vi "filter_test.vi"(9 "Throughput-1":i16=17, 10 "reset":bool, 11 "input valid":bool) -> (0 "run?":bool, 1 "ready for input":bool, 2 "load":bool, 3 "output valid":bool, 5 "reset for cu":bool, 7 "idx":i16)   [LabVIEW 2021]
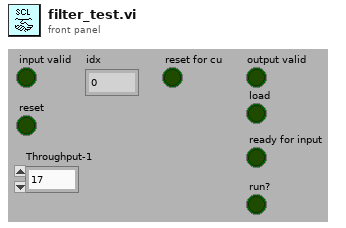
[diagram p1: front panel]
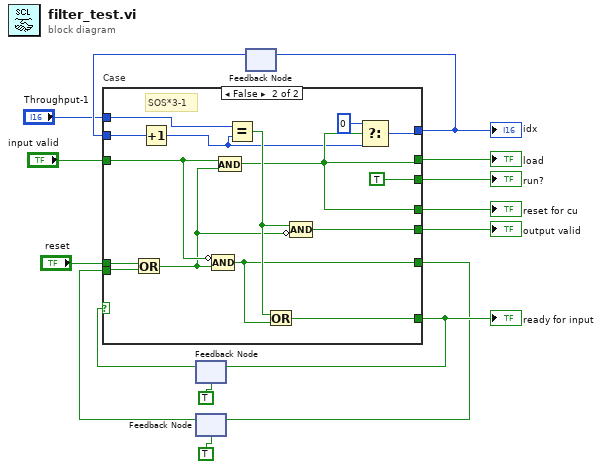
[diagram p0: block diagram]
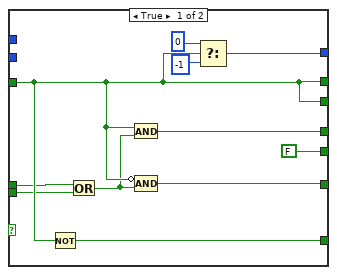
[diagram p2: hidden frame]
diagram:
  n1 = feedback #1(TRUE) -> (w15:bool)
  n2 = feedback #2(TRUE) -> (w2:bool)
  n3 = feedback #3() -> (w8:i16)  [unwired: 1 out]
  n4 = case "Case" shown="False" w15 {
    tunnel: "input valid" -> [w20 w34]
    tunnel: [w20 TRUE ("input valid")] -> w14
    tunnel: [w20 w31] -> w13
    tunnel: [w24 w29] -> w7
    tunnel: w8 -> [_ w41]
    tunnel: [FALSE w39] -> w12
    tunnel: [w22 w38] -> w10
    tunnel: "reset" -> [w17 w35]
    tunnel: [w19 w31] -> w5
    tunnel: [w21 w32] -> w3
    tunnel: w2 -> [w18 w36]
    tunnel: "Throughput-1" -> [_ w27]
    frame True {
      n5 = Not(x=w20) -> (.not. x?=w22:bool)
      n6 = Or(x=w17, y=w18) -> (x .or. y?=w16:bool)
      n7 = And(x=w20, y=w16) -> (x .and. y?=w19:bool)
      n8 = Compound Arithmetic op=AND(invert w20, w16) -> (w21:bool)
      n9 = Select(t=i16 0, s=w20, f=i16 -1) -> (s? t:f=w24:i16)
    }
    frame False {
      # "SOS*3-1"
      n10 = Or(x=w35, y=w36) -> (x .or. y?=w33:bool)
      n11 = Increment(x=w41) -> (x+1=w30:i16)
      n12 = Compound Arithmetic op=AND(invert w34, w33) -> (w32:bool)
      n13 = And(x=w34, y=w33) -> (x .and. y?=w31:bool)
      n14 = Equal?(x=w27, y=w30) -> (x = y?=w37:bool)
      n15 = Or(x=w37, y=w32) -> (x .or. y?=w38:bool)
      n16 = Compound Arithmetic op=AND(w37, invert w33) -> (w39:bool)
      n17 = Select(t=i16 0 ("y"), s=w31, f=w30) -> (s? t:f=w29:i16)
    }
  }
  "run?" <- w14
  "ready for input" <- w10
  "load" <- w13
  "output valid" <- w12
  "idx" <- w7
  "reset for cu" <- w5
  n18 = feedback-in #1(w10) -> ()
  n19 = feedback-in #2(w3) -> ()
  n20 = feedback-in #3(w7) -> ()
